vi "calcDerivedDisplacementPrevious.vi"(8 "error in (no error)":errorcluster, 11 "StiffnessMonitor in":refnum<class "StiffnessMonitor.lvclass">) -> (0 "error out":errorcluster, 3 "StiffnessMonitor out":refnum<class "StiffnessMonitor.lvclass">)   [LabVIEW 2013, in "StiffnessMonitor.lvclass"]
uses:
  StiffnessMonitor.lvclass
  StiffnessMonitor.lvclass/StiffnessMonitor.ctl
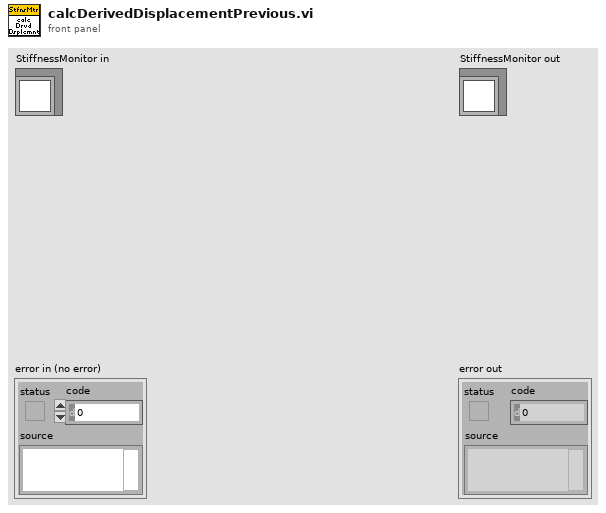
[diagram p1: front panel]
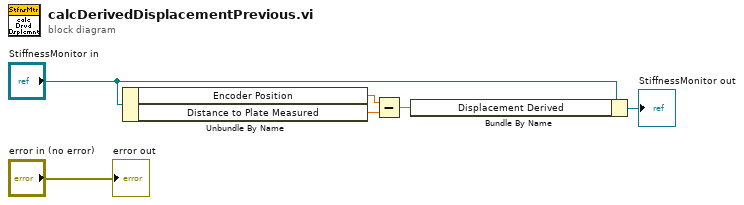
[diagram p0: block diagram]
diagram:
  n1 = Unbundle By Name("StiffnessMonitor in") -> ("Encoder Position"=w5:dbl[unit], "Distance to Plate Measured"=w4:dbl[unit])
  n2 = Subtract(x=w5, y=w4) -> (x-y=w3:dbl[unit])
  n3 = Bundle By Name(cluster="StiffnessMonitor in", "Displacement Derived"=w3) -> (→"StiffnessMonitor out":refnum<class "StiffnessMonitor.lvclass">)
  "error out" <- "error in (no error)"
